vi "SGEN_DC_33521A.vi"(4 "Output Impedance (50 Ohm)":dbl=inf format="%#_13g", 6 "Enable Output (T: Enable)":bool=TRUE, 8 "error in (no error)":errorcluster, 10 "DC Offset (0 V)":dbl, 11 "VISA_SGEN":refnum<visa-resource-name>="USB0::0x0957::0x1607::MY50001293::INSTR") -> (0 "error out":errorcluster)   [LabVIEW 2019]
uses:
  <userlib>/_TI-LA/Instr Drivers/Signal Generator/3352x/Driver/Base/Agilent 3352X Series.lvlib
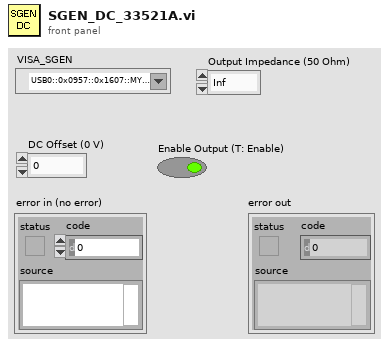
[diagram p1: front panel]
types:
  T1 = enum16{"Numeric", "High Z", "Minimum", "Maximum", "Default"}
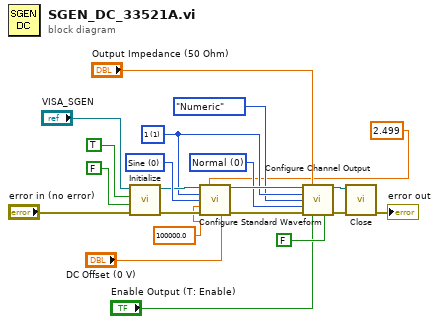
[diagram p0: block diagram]
diagram:
  w3 = 0 items=["Normal", "Gated"] ("Output State (0: Normal)")
  w14 = 1 items=["1"=1, "2"=2] ("Channel (1: 1)")
  w21 = 0 items=["Sine"=0, "Square"=1, "Ramp"=2, "Noise"=3, "DC"=4, "Triangle"=5, "Pulse"=6, "Sinc"=11, "D-Lorentz"=12, "Gaussian"=13, "Expo Fall"=14, "Expo Rise"=15, "Haversine"=16] ("Waveform Function (0: Sine)")
  n1 = call <userlib>:"Initialize.vi"("error in (no error)"="error in (no error)", "Reset (Enable)"=FALSE, "ID Query (Enable)"=TRUE, "VISA resource name"="VISA_SGEN") -> ("error out"=w15:errorcluster, "VISA resource name out"=w16:refnum<visa-resource-name>)  [unwired: 6 in]
  n2 = call <userlib>:"Configure Standard Waveform.vi"("VISA resource name"=w16, "Amplitude (0.1 Vpp)"=2.499, "Channel (1: 1)"=w14, "Waveform Function (0: Sine)"=w21, "Frequency/Sample Rate/Bandwidth (1000 Hz)"=100000.0, "error in (no error)"=w15, "DC Offset (0 V)"="DC Offset (0 V)") -> ("VISA resource name out"=w18:refnum<visa-resource-name>, "error out"=w17:errorcluster)  [unwired: 7 in]
  n3 = call <userlib>:"Configure Channel Output.vi"("VISA resource name"=w18, "Output Impedance (50 Ohm)"="Output Impedance (50 Ohm)", "Channel (1: 1)"=w14, "Output Impedence Mode (0: Numeric)"=T1."Numeric", "Output State (0: Normal)"=w3, "error in (no error)"=w17, "Enable Output (T: Enable)"="Enable Output (T: Enable)", "Enable Voltage Limit (T: Enable)"=FALSE) -> ("VISA resource name out"=w20:refnum<visa-resource-name>, "error out"=w19:errorcluster)  [unwired: 6 in]
  n4 = call <userlib>:"Close.vi"("error in (no error)"=w19, "VISA resource name"=w20) -> ("error out"=→"error out":errorcluster)  [unwired: 9 in]
